vi "GlobalVariables.vi"() -> ()   [LabVIEW 2014]
panel:
  out "Spec Vac":string
  out "SC Vac":string
  out "BL Vac":string
  out "Spectrograph 2 (High Vac)":string
  out "Spectrograph Vacuum":string
  out "Scat. Chamber":string
  out "Scatt TC (Torr)":string
  out "Beamline":string
  out "Beamline TC1 (Torr) 2":string
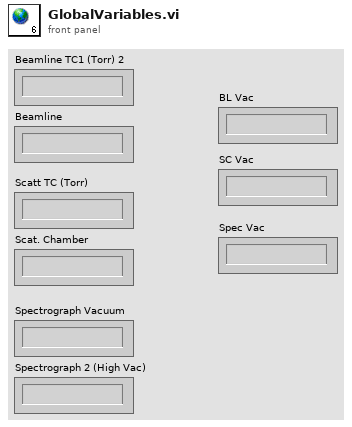
[diagram p1: front panel]
diagram:
